vi "Write Defaults File.vi"(0 "DirPath3":path=path "C:/SixBeam/Movies", 1 "DirPath2":path=path "C:/SixBeam/Images", 2 "DirPath1":path=path "C:/SixBeam/SixBeam.llb", 3 "DefaultFilename":string="Pole4.dft", 4 "MiscPath10":path=path "<not a path10>", 5 "MiscPath9":path=path "<not a path9", 6 "MiscPath8":path=path "<not a path8>", 7 "MiscPath7":path=path "<not a path7>", 8 "DirPath4":path=path "C:/SixBeam/<empty4>", 9 "MiscPath6":path=path "<not a path6>", 10 "DirPath5":path=path "C:/SixBeam/<empty5>", 11 "MiscPath5":path=path "<not a path5>", 12 "String1":string="SixBeam.set", 13 "MiscPath4":path=path "<not a path4>", 14 "String2":string="SixBeam.cal", 15 "MiscPath3":path=path "<not a path3>", 16 "String3":string="SixBeam.pdb", 17 "MiscPath2":path=path "<not a path2>", 18 "String4":string="Unused.4", 19 "MiscPath1":path=path "<not a path1>", 20 "String5":string="Unused.5", 21 "BooleanArray":bool[](array[boolean])=[FALSE], 22 "IntegerArray1":i32[](array[numeric])=[0], 24 "IntegerArray2":i32[](array[numeric])=[0], 25 "RealArray1":dbl[](array[numeric])=[0.0] format="%.2f", 26 "RealArray2":dbl[](array[numeric])=[0.0] format="%.2f", 27 "StringArray":string[](array[string])=["<empty string>"]) -> ()   [LabVIEW 2013]
doc: "This vi writes program default values to an ASCII file. Many different types of variables can be output (see the connector listing for details). Single parameters are written to a single line; arrays are written as a single line with each array element separated by commas. Each line is terminated with a carriage return & linefeed. The vi uses the \"Write Chars to File.vi\" which creates a new file if one is not found, or writes over an existing one. The filename is input at \"DefaultFilename\" and the file is written to the directory from which this vi is run. AutoCon, 11/98"
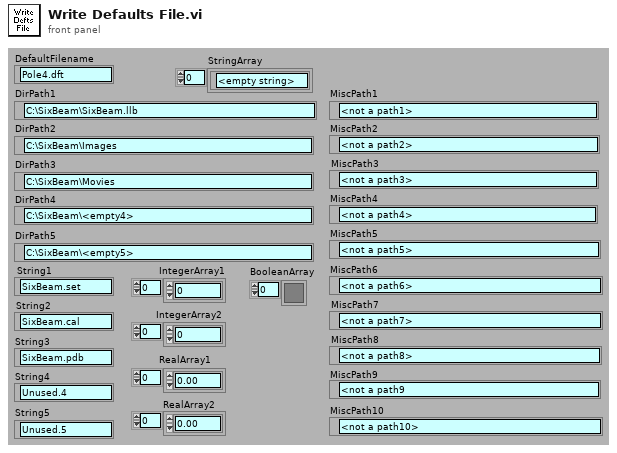
[diagram p1: front panel]
types:
  T1 = enum16{"String", "I32", "Sgl", "Dbl", "Boolean", "U32", "Path"}
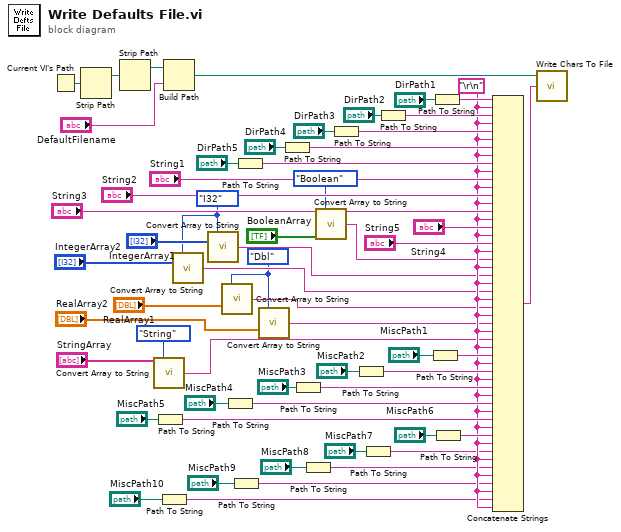
[diagram p0: block diagram]
diagram:
  w3 = T1."Dbl" ("Type")
  w2 = T1."I32" ("Type")
  w27 = "\r\n"
  n1 = Current VI's Path() -> (path=w58:path)
  n2 = Strip Path(path=w58) -> (stripped path=w57:path)  [unwired: 1 out]
  n3 = Strip Path(path=w57) -> (stripped path=w56:path)  [unwired: 1 out]
  n4 = call "Convert Array to String.vi"("StringArrayIn"="StringArray", "Type"=T1."String") -> ("StringOut"=w5:string)  [unwired: 13 in]
  n5 = Path To String(path="MiscPath5") -> (string=w30:string)
  n6 = Path To String(path="MiscPath10") -> (string=w19:string)
  n7 = Build Path(base path=w56, name or relative path="DefaultFilename") -> (appended path=w18:path)
  n8 = call "Convert Array to String.vi"("Type"=w2, "I32ArrayIn"="IntegerArray2") -> ("StringOut"=w11:string)  [unwired: 13 in]
  n9 = call "Convert Array to String.vi"("Type"=w2, "I32ArrayIn"="IntegerArray1") -> ("StringOut"=w14:string)  [unwired: 13 in]
  n10 = call "Convert Array to String.vi"("Type"=w3, "DblArrayIn"="RealArray1") -> ("StringOut"=w10:string)  [unwired: 13 in]
  n11 = Path To String(path="MiscPath4") -> (string=w32:string)
  n12 = Path To String(path="MiscPath9") -> (string=w21:string)
  n13 = Path To String(path="DirPath5") -> (string=w45:string)
  n14 = call "Convert Array to String.vi"("Type"=w3, "DblArrayIn"="RealArray2") -> ("StringOut"=w8:string)  [unwired: 13 in]
  n15 = Path To String(path="DirPath4") -> (string=w47:string)
  n16 = Path To String(path="MiscPath3") -> (string=w34:string)
  n17 = Path To String(path="MiscPath8") -> (string=w23:string)
  n18 = call "Convert Array to String.vi"("Type"=T1."Boolean", "BooleanArrayIn"="BooleanArray") -> ("StringOut"=w16:string)  [unwired: 13 in]
  n19 = Path To String(path="DirPath3") -> (string=w49:string)
  n20 = Path To String(path="MiscPath2") -> (string=w36:string)
  n21 = Path To String(path="MiscPath7") -> (string=w25:string)
  n22 = Path To String(path="DirPath2") -> (string=w53:string)
  n23 = Path To String(path="MiscPath1") -> (string=w38:string)
  n24 = Path To String(path="DirPath1") -> (string=w55:string)
  n25 = Path To String(path="MiscPath6") -> (string=w28:string)
  n26 = Concatenate Strings(w55, w27, w53, w27, w49, w27, w47, w27, w45, w27, "String1", w27, "String2", w27, "String3", w27, "String4", w27, "String5", w27, w16, w27, w14, w27, w11, w27, w10, w27, w8, w27, w5, w27, w38, w27, w36, w27, w34, w27, w32, w27, w30, w27, w28, w27, w25, w27, w23, w27, w21, w27, w19, w27) -> (w17:string)
  n27 = call "Write Chars To File.vi"("character string"=w17, "file path (dialog if empty)"=w18) -> ()  [unwired: 3 in, 1 out]
